vi "fgv_data.vi"(7 "cmd":T2, 8 "error in":errorcluster, 11 "action":T1=enum."on") -> (0 "error out":errorcluster, 3 "queue out":refnum<queue>)   [LabVIEW 2019]
uses:
  _ctrl/create-rw-close.ctl
  _ctrl/DSP_action.ctl
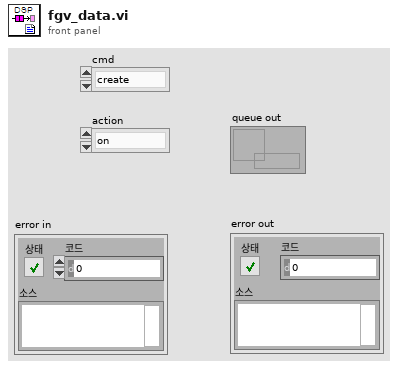
[diagram p1: front panel]
types:
  T1 = typedef "DSP_action.ctl" = enum16{"False", "cont", "on", "off", "discont", "protection", "preread", "level", "read", "stop", "exit"}
  T2 = typedef "create-rw-close.ctl" = enum16{"create", "write", "read", "delete", "close"}
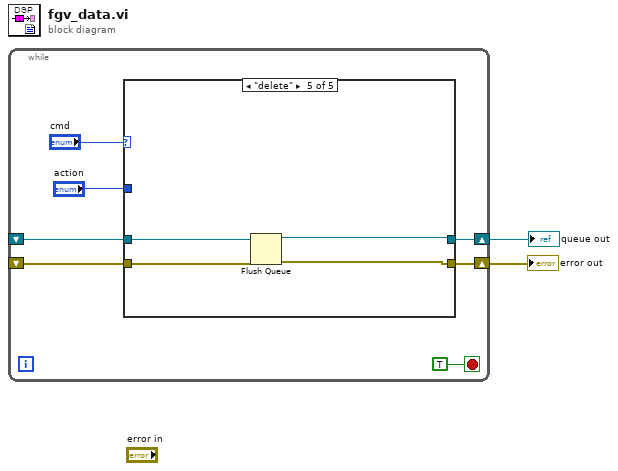
[diagram p0: block diagram]
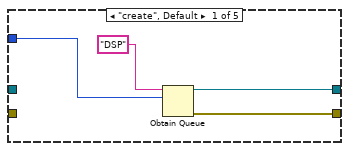
[diagram p2: hidden frame]
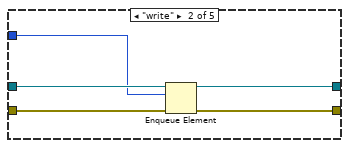
[diagram p3: hidden frame]
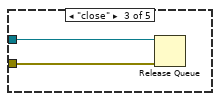
[diagram p4: hidden frame]
diagram:
  n1 = while {
    shift-right: [w5] -> w1
    shift-left: _ -> [w7]
    shift-right: [w6] -> w2
    shift-left: _ -> [w8]
    stop <- TRUE stop-if-true
    n2 = case shown="\"delete\"" "cmd" {
      tunnel: w8 -> [_ w18 w20 w22 w25]
      tunnel: w7 -> [_ w17 w19 w21 w26]
      tunnel: "action" -> [w13 w16 _ _ _]
      tunnel: [w11 w15 _ w22 w24] -> w6
      tunnel: [w10 w14 _ w21 w23] -> w5
      frame "create", Default {
        n3 = Obtain Queue(name (unnamed)="DSP" ("이름(이름없음)"), element data type=w13) -> (queue out=w10:refnum<queue>, error out=w11:errorcluster)  [unwired: 3 in, 1 out]
      }
      frame "write" {
        n4 = Enqueue Element(queue=w17, element=w16, error in (no error)=w18) -> (queue out=w14:refnum<queue>, error out=w15:errorcluster)  [unwired: 1 in, 1 out]
      }
      frame "close" {
        n5 = Release Queue(queue=w19, error in (no error)=w20) -> ()  [unwired: 1 in, 3 out]
      }
      frame "read" {
      }
      frame "delete" {
        n6 = Flush Queue(queue=w26, error in (no error)=w25) -> (queue out=w23:refnum<queue>, error out=w24:errorcluster)  [unwired: 1 out]
      }
    }
  }
  "error out" <- w2
  "queue out" <- w1
